vi "VIinClass.vi"() -> ()   [LabVIEW 2023, in "ClassForClassMemberCall.lvclass"]
uses:
  ClassForClassMemberCall.lvclass
panel:
  out "Result":dbl
  in  "Y":dbl
  in  "X":dbl
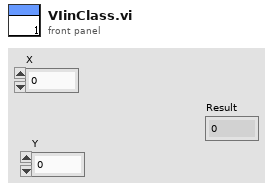
[diagram p1: front panel]
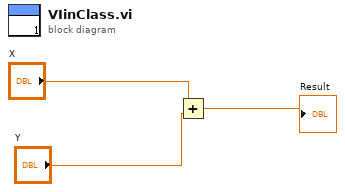
[diagram p0: block diagram]
diagram:
  n1 = Add(x="X", y="Y") -> (x+y=→"Result":dbl)
